vi "Return.vi"(8 "error in (no error)":errorcluster, 10 "Tx String":string, 11 "Parrot in":refnum<class "Parrot.lvclass">) -> (0 "error out":errorcluster, 3 "Parrot out":refnum<class "Parrot.lvclass">)   [LabVIEW 2016, in "Parrot.lvclass"]
doc: "--\nCopyright © 2017 Composed SystemsI All rights reserved.\n\nAuthor: Jon McBee <jon.mcbee@composed.io>\n\nThis library is provided \"AS IS\" ,WITHOUT WARRANTIES OR\nCONDITIONS OF ANY KIND, either express or implied.\n\nComposed Systems -- composed.io\n\nStream 0.0.1.1\nJon McBee - Composed Systems\nCopyright (c) 2017, Composed Systems"
uses:
  <userlib>/Composed Systems/Stream/Sandbox/Async Actor Test/Parrot Actor/Parrot.lvclass
  C:/Program Files (x86)/National Instruments/LabVIEW 2016/user.lib/Composed Systems/Stream/Mediator/Classes/Mediated Asynchronous Actor/Mediated Asynchronous Actor.lvclass
  <userlib>/Composed Systems/Stream/Mediator/Classes/Message String/Message String.lvclass
  C:/Program Files (x86)/National Instruments/LabVIEW 2016/user.lib/Composed Systems/Stream/Mediator/Classes/Message Interface/Message Interface.lvclass
  <userlib>/Composed Systems/Stream/Sandbox/Async Actor Test/Parrot Actor/Parrot.lvclass/Parrot.ctl
  <userlib>/Composed Systems/Stream/Mediator/Classes/Message Transport Queue/Message Transport Queue.lvclass
  <userlib>/Composed Systems/Stream/Mediator/Classes/Mediated Asynchronous Actor/Mediated Asynchronous Actor.lvclass
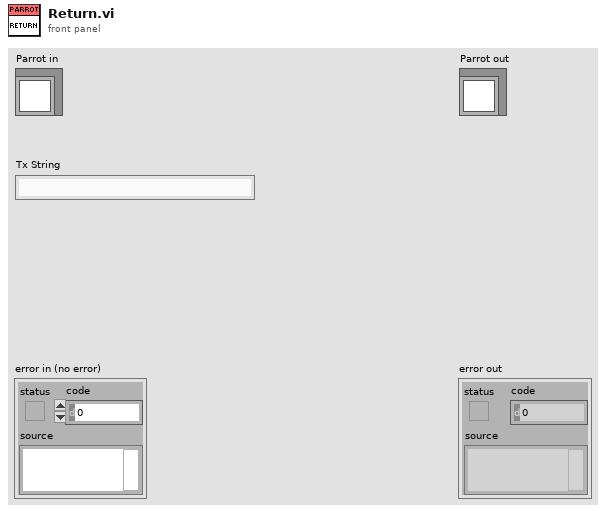
[diagram p1: front panel]
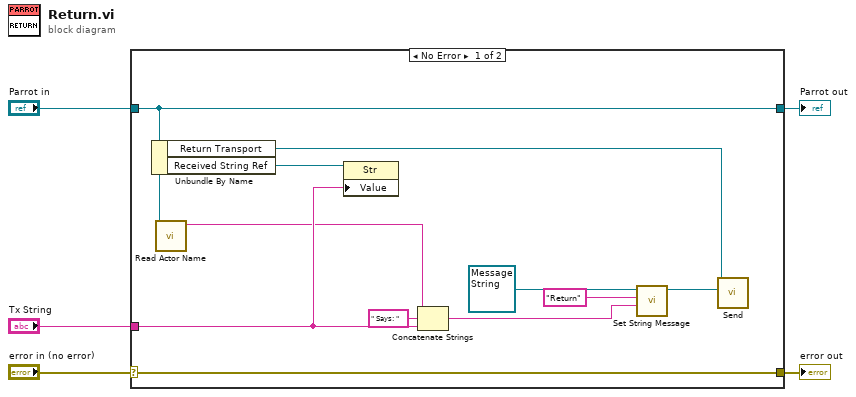
[diagram p0: block diagram]
diagram:
  n1 = case shown="No Error" "error in (no error)" {
    selector: "error in (no error)" -> [w16 w18]
    tunnel: [w16 w18] -> w4
    tunnel: [w7 w17] -> w2
    tunnel: "Parrot in" -> [w7 w17]
    tunnel: "Tx String" -> [w8 _]
    frame No Error {
      n2 = Unbundle By Name(w7) -> ("Return Transport"=w11:refnum<class "Message Transport Queue.lvclass">, "Received String Ref"=w9:refnum<vi>)
      n3 = call <userlib>:"Read Actor Name.vi"("Mediated Asynchronous Actor in"=w7) -> ("Actor Name"=w6:string)  [unwired: 10 in]
      n4 = property class="Str"(reference=w9, "Value"=w8) -> ()  [unwired: 1 in, 2 out]
      n5 = Concatenate Strings(w6, " Says: " ("string"), w8) -> (w13:string)
      n6 = call <userlib>:"Set String Message.vi"("Value"=w13, "Name"="Return", "Message String in"=refnum<class "Message String.lvclass"> refnum) -> ("Message String out"=w10:refnum<class "Message String.lvclass">)  [unwired: 7 in, 1 out]
      n7 = call-dynamic "Send.vi"("Message"=w10, "Message Transport Queue in"=w11) -> ()  [unwired: 7 in, 3 out]
    }
    frame Error {
    }
  }
  "error out" <- w4
  "Parrot out" <- w2
